vi "worksheet ignore errors.vi"(8 "error in (no error)":errorcluster, 9 "range":string, 10 "type":u8, 11 "worksheet":u32) -> (0 "error out":errorcluster, 3 "function return":u32(ring))   [LabVIEW 8.6]
doc: "lxw_error worksheet_ignore_errors(lxw_worksheet worksheet, uint8_t type, const char *range);"
uses:
  pending_lvxlsxwriter/xlsxwriter.dll
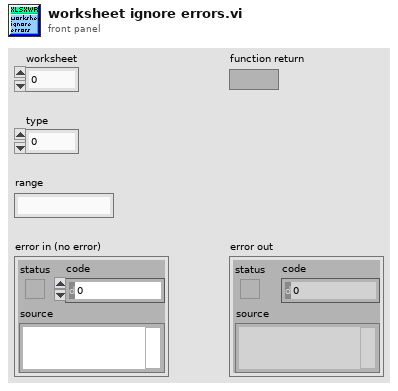
[diagram p1: front panel]
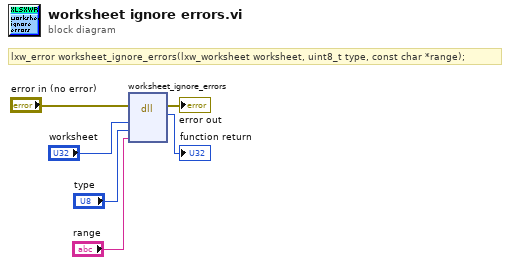
[diagram p0: block diagram]
diagram:
  # "lxw_error worksheet_ignore_errors(lxw_worksheet worksheet, uint8_t type, const char *range);"
  n1 = dll-call lib="C:/Users/WDAGUtilityAccount/Desktop/pending_lvxlsxwriter/xlsxwriter.*" fn="worksheet_ignore_errors"(error in="error in (no error)", "worksheet"="worksheet", "type"="type", "range"="range") -> (error out=→"error out":errorcluster, →"function return":u32)  [unwired: 5 in, 1 out]
